vi "HV_Grid Viewer.vi"() -> ()   [LabVIEW 2018]
uses:
  SPD Stand/typedefs/SPD.Meas Result.ctl
panel:
  out "Waveform Graph":dbl[][](graph)
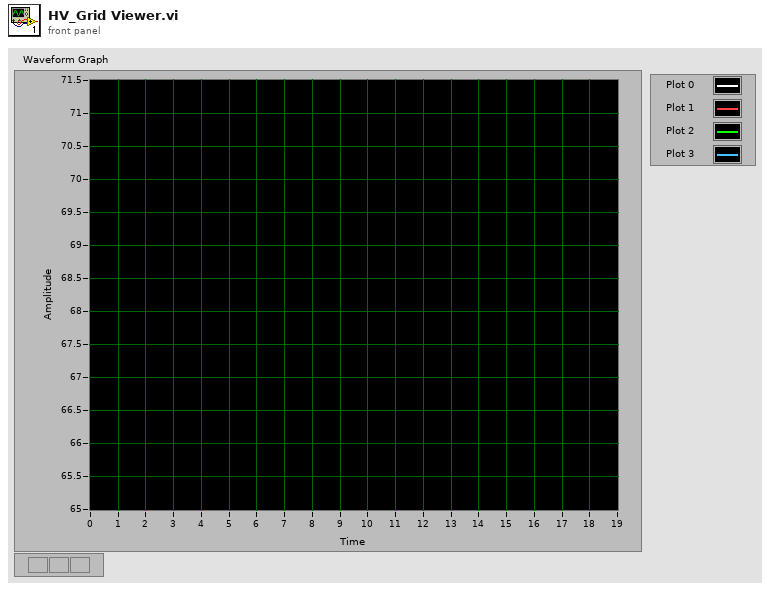
[diagram p1: front panel]
types:
  T1 = typedef "SPD.Meas Result.ctl" = cluster{"HV_Bias":dbl[][], "Stb_code":dbl[], "Temprature":dbl[], "Data":dbl[][][][]}
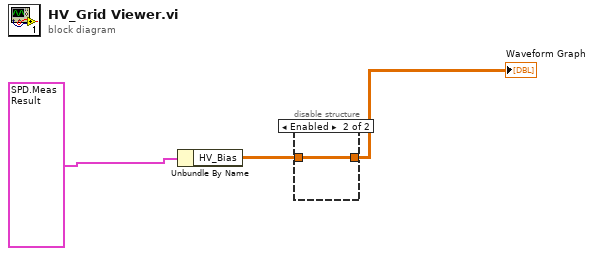
[diagram p0: block diagram]
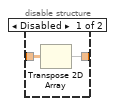
[diagram p2: hidden frame]
diagram:
  n1 = Unbundle By Name(T1 {"HV_Bias"=array63x20[1260 elements], "Stb_code"=[0.0, 51.0, 102.0, 153.0, 204.0, 255.0, 306.0, 357.0, 408.0, 459.0, 510.0, 561.0, 612.0, 663.0, 714.0, 765.0, 816.0, 867.0, 918.0, 969.0, 1020.0], "Temprature"=[-50.0, -47.5, -45.0], "Data"=[]} ("SPD.Result")) -> ("HV_Bias"=w3:dbl[][])
  n2 = disable-structure shown="Enabled" {
    disable-tunnel: w3 -> [w5 w6]
    disable-tunnel: [w4 w6] -> w2
    frame Disabled {
      n3 = Transpose 2D Array(2D array=w5) -> (transposed array=w4:dbl[][])
    }
    frame Enabled {
    }
  }
  "Waveform Graph" <- w2
